vi "SUB_SFCS_CHK_RFPI_IPEI_Unique.vi"(0 "URL":string, 1 "LINE":string, 3 "OP_ID":string, 5 "SN":string, 7 "Assembly_True_FLASE":u8, 9 "Stage":string, 11 "RFID_content":string, 12 "STATION":string, 14 "SFCS_RFID_CATGORY":string) -> (4 "PASS?":bool, 15 "output param":string)   [LabVIEW 2011]
uses:
  IPEI_RFPI.dll
panel:
  out "length":i32
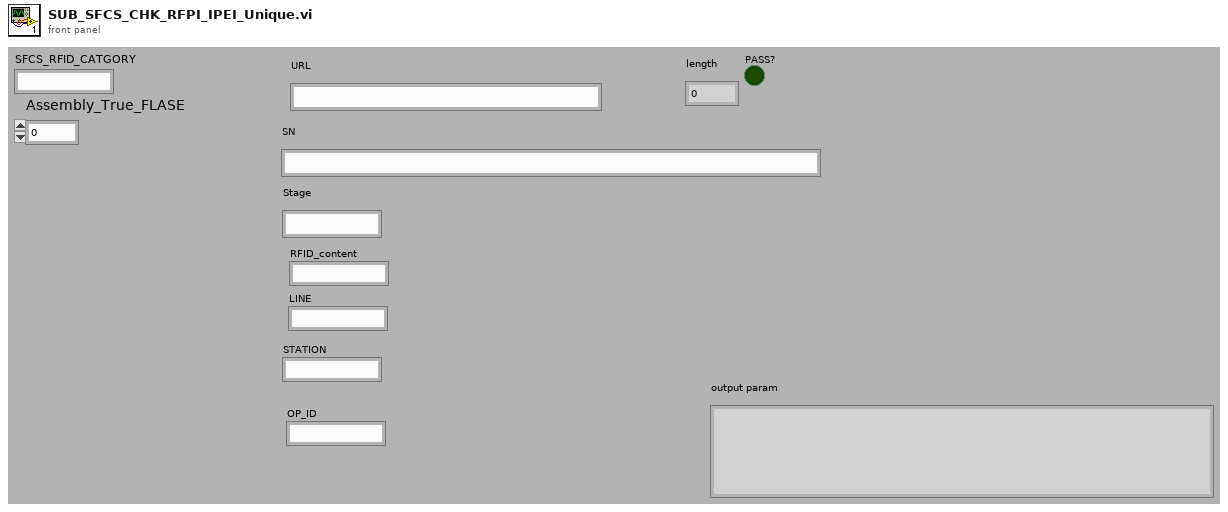
[diagram p1: front panel]
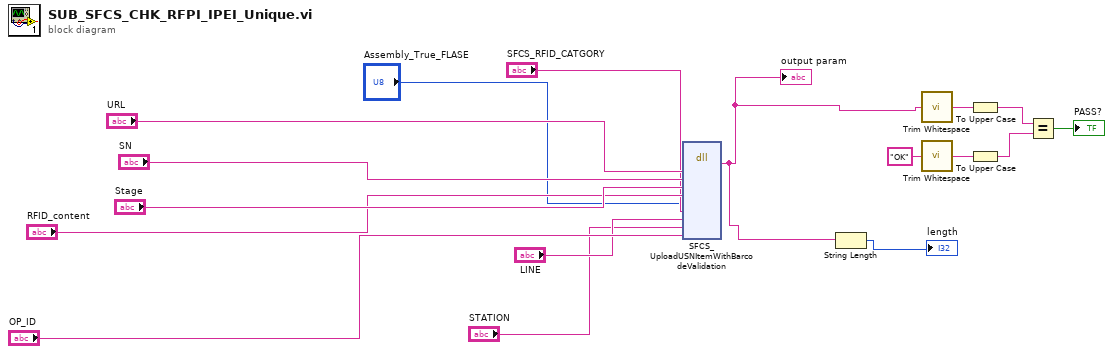
[diagram p0: block diagram]
diagram:
  n1 = dll-call lib="D:/Konftel_Project/IPEI_RFPI.dll" fn="SFCS_UploadUSNItemWithBarcodeValidation"("URL"="URL", "SN"="SN", "Stage"="Stage", "RFID_content"="RFID_content", "Assembly_True_FLASE"="Assembly_True_FLASE", "CAT"="SFCS_RFID_CATGORY", "LINE"="LINE", "STATION"="STATION", "OP_ID"="OP_ID") -> (w8:string)  [unwired: 12 in, 2 out]
  "output param" <- w8
  n2 = String Length(string=w8) -> (length=→"length":i32)
  n3 = call <vilib>:"Trim Whitespace.vi"("string"=w8) -> ("trimmed string"=w9:string)  [unwired: 1 in]
  n4 = call <vilib>:"Trim Whitespace.vi"("string"="OK") -> ("trimmed string"=w7:string)  [unwired: 1 in]
  n5 = To Upper Case(1:w9) -> (0:w5:string)
  n6 = To Upper Case(1:w7) -> (0:w4:string)
  n7 = Equal?(x=w5, y=w4) -> (x = y?=→"PASS?":bool)
